vi "lv2012 - Bind Shared Variables with EPICS subVI.vi"(11 "vi path":path=path "C:/Users/kvlb23/Documents/KVLB Test Area/Research/data binding/lv2012 - SubVI 2.vi") -> (0 "error out":errorcluster)   [LabVIEW 2012]
uses:
  <vilib>/variable/tagger/epicsserver/API/internal/Undeploy EPICS Server (By Ref).vi
  Labview Modules/Common/Utilities/Equal.llb/Equal - Variant.vi
  Labview Modules/Common/Utilities/Equal.llb/Equal - String.vi
  <vilib>/variable/tagger/epicsserver/API/internal/EPICSServerClass/EPICSServer.lvclass
  <vilib>/lvdsc/NI_DSC.lvlib
  <vilib>/variable/tagger/epicsserver/API/NI_EPICS_Server.lvlib
panel:
  in  "Stop Button":bool
  in  "error in (no error)":errorcluster
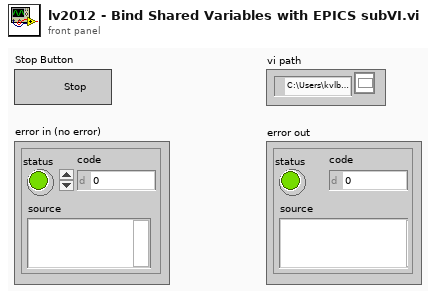
[diagram p1: front panel]
types:
  T1 = enum32{"No PSP", "Read", "Write", "Write & Read"}
  T2 = enum32{"u32BitField", "bool", "double", "string", "int8", "uint8", "int16", "uint16", "int32", "uint32", "int64", "uint64", "single", "double waveform", "int16 waveform", "array of boolean", "array of int8", "array of uint8", "array of int16", "array of uint16", "array of int32", "array of uint32", "array of int64", "array of uint64", "array of single", "array of double", "array of double waveform", "array of int16 waveform", "array of string", "variant", "timestamp", "fixed point", "custom"}
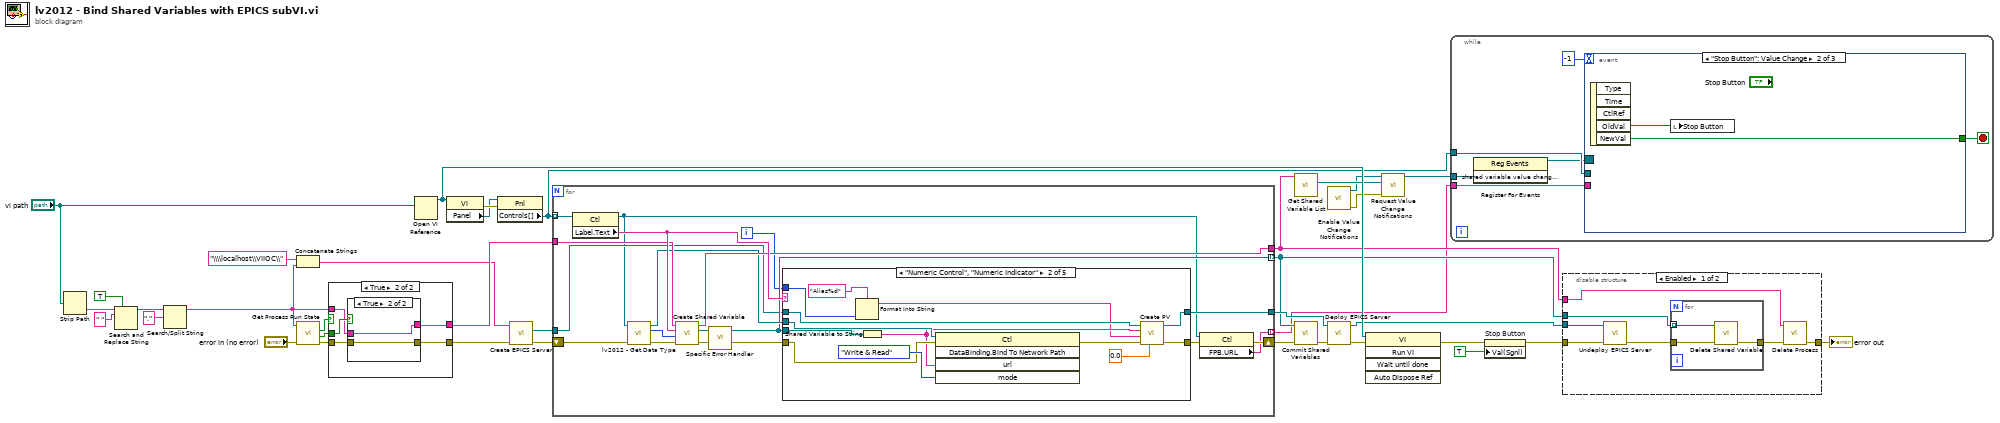
[diagram p0: block diagram]
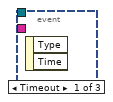
[diagram p2: hidden frame]
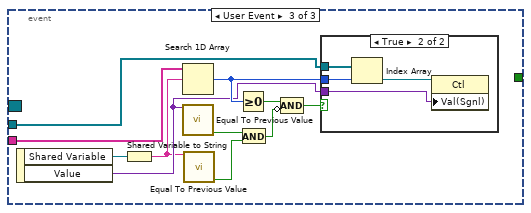
[diagram p3: hidden frame]
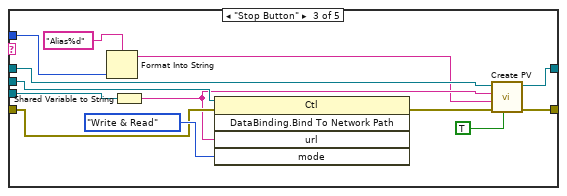
[diagram p7: hidden frame]
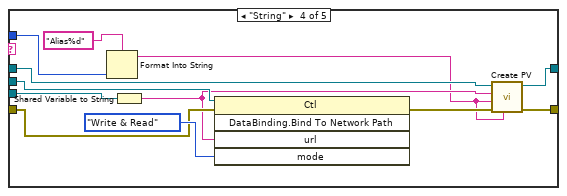
[diagram p8: hidden frame]
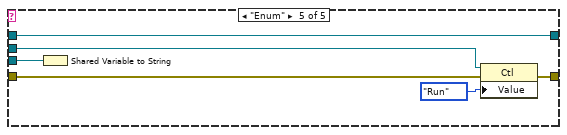
[diagram p9: hidden frame]
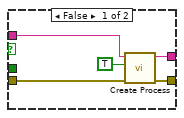
[diagram p10: hidden frame]
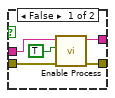
[diagram p11: hidden frame]
diagram:
  n1 = Strip Path(path="vi path") -> (name=w17:string)  [unwired: 1 out]
  n2 = Search and Replace String(replace all?=TRUE ("replace all? (F)"), input string=w17, search string=" ") -> (result string=w14:string)  [unwired: 5 in, 3 out]
  n3 = Search/Split String(string=w14, search string/char (-)="." ("regular expression")) -> (substring before match=w12:string)  [unwired: 1 in, 2 out]
  n4 = Concatenate Strings("\\\\localhost\\VIIOC\\" ("format string"), w12) -> (w18:string)
  n5 = call <vilib>:"Get Process Run State.vi"("error in (no error)"="error in (no error)", "process name"=w12) -> ("error out"=w34:errorcluster, "running?"=w33:bool, "exists?"=w36:bool)  [unwired: 6 in, 1 out]
  n6 = case shown="True" w36 {
    tunnel: w12 -> [w42 w46]
    tunnel: [w39 w44] -> w29
    tunnel: w34 -> [w41 w45]
    tunnel: [w38 w43] -> w27
    tunnel: w33 -> [_ w47]
    frame False {
      n7 = call <vilib>:"Create Process.vi"("error in (no error)"=w41, "run?"=TRUE, "process name"=w42) -> ("error out"=w38:errorcluster, "process name out"=w39:string)  [unwired: 7 in]
    }
    frame True {
      n8 = case shown="True" w47 {
        tunnel: w46 -> [w51 w54]
        tunnel: w45 -> [w50 w53]
        tunnel: [w49 w54] -> w44
        tunnel: [w48 w53] -> w43
        frame False {
          n9 = call <vilib>:"Enable Process.vi"("error in (no error)"=w50, "run?"=TRUE, "process name"=w51) -> ("error out"=w48:errorcluster, "process name out"=w49:string)  [unwired: 7 in]
        }
        frame True {
        }
      }
    }
  }
  n10 = Open VI Reference(vi path="vi path") -> (vi reference=w30:refnum<vi>)  [unwired: 5 in, 1 out]
  n11 = property class="VI"(reference=w30) -> (error out=w32:errorcluster, "Panel"=w31:refnum<vi>)  [unwired: 1 in, 1 out]
  n12 = property class="Pnl"(reference=w31, error in=w32) -> ("Controls[]"=w6:refnum<vi>[])  [unwired: 2 out]
  n13 = call <vilib>:"Create EPICS Server.vi"("error in (no error)"=w27, "EPICS Server URL in"=w18) -> ("error out"=w26:errorcluster, "EPICS Server ref"=w25:refnum<data-value>)  [unwired: 7 in, 1 out]
  n14 = for {
    tunnel: w6 -> [w72] mode=indexing
    shift-right: [w57] -> w22
    shift-left: w26 -> [w67]
    tunnel: w29 -> [w70]
    tunnel: [w69] -> w7
    tunnel: [w63] -> w23 mode=indexing
    tunnel: [w61] -> w28
    tunnel: w25 -> [w62]
    tunnel: [w55] -> w5 mode=indexing
    i -> [w60]
    n15 = property class="Ctl"(reference=w72) -> (reference out=w56:refnum<vi>, "Label.Text"=w71:string)  [unwired: 1 in, 1 out]
    n16 = call "lv2012 - Get Data Type.vi"("error in (no error)"=w67, "Control in"=w56) -> ("error out"=w66:errorcluster, "data type"=w65:T2, "Control out"=w64:refnum<vi>)  [unwired: 7 in]
    n17 = call <vilib>:"Create Shared Variable.vi"("error in (no error)"=w66, "data type"=w65, "shared variable name"=w71, "process name"=w70) -> ("error out"=w59:errorcluster, "shared variable"=w63:refnum<k21>, "process name out"=w69:string)  [unwired: 5 in]
    n18 = call "Specific Error Handler"("Error to Check"=w59) -> ("error out"=w68:errorcluster)  [unwired: 11 in, 3 out]
    n19 = case shown="\"Numeric Control\", \"Numeric Indicator\"" w71 {
      tunnel: w64 -> [_ w86 w99 w111 w116]
      tunnel: [w74 w81 w94 w106 w118] -> w58
      tunnel: w68 -> [w74 w85 w98 w110 w117]
      tunnel: w63 -> [_ w80 w93 w105 w113]
      tunnel: w62 -> [w73 w84 w97 w109 w114]
      tunnel: [w73 w83 w96 w108 w114] -> w61
      tunnel: w60 -> [_ w77 w91 w103 _]
      frame Default {
      }
      frame "Numeric Control", "Numeric Indicator" {
        n20 = Format Into String(format string="Alias%d", w77) -> (resulting string=w75:string)  [unwired: 2 in, 1 out]
        n21 = Shared Variable to String(1:w80) -> (0:w79:string)
        n22 = invoke on="Invoke Node" class="Ctl" method="DataBinding.Bind To Network Path"(reference=w86, error in=w85, "url"=w79, "mode"=T1."Write & Read" ("Data Binding:Mode")) -> (error out=w82:errorcluster)  [unwired: 1 in, 4 out]
        n23 = call <vilib>:"Create PV.vi"("data type"=0.0, "error in (no error)"=w82, "PV name"=w75, "variable path"=w79, "EPICS Server ref in"=w84) -> ("error out"=w81:errorcluster, "EPICS Server ref out"=w83:refnum<data-value>)  [unwired: 5 in]
      }
      frame "Stop Button" {
        n24 = Format Into String(format string="Alias%d", w91) -> (resulting string=w88:string)  [unwired: 2 in, 1 out]
        n25 = Shared Variable to String(1:w93) -> (0:w92:string)
        n26 = invoke on="Invoke Node" class="Ctl" method="DataBinding.Bind To Network Path"(reference=w99, error in=w98, "url"=w92, "mode"=T1."Write & Read" ("Data Binding:Mode")) -> (error out=w95:errorcluster)  [unwired: 1 in, 4 out]
        n27 = call <vilib>:"Create PV.vi"("data type"=TRUE, "error in (no error)"=w95, "PV name"=w88, "variable path"=w92, "EPICS Server ref in"=w97) -> ("error out"=w94:errorcluster, "EPICS Server ref out"=w96:refnum<data-value>)  [unwired: 5 in]
      }
      frame "String" {
        n28 = Format Into String(format string="Alias%d", w103) -> (resulting string=w101:string)  [unwired: 2 in, 1 out]
        n29 = Shared Variable to String(1:w105) -> (0:w104:string)
        n30 = invoke on="Invoke Node" class="Ctl" method="DataBinding.Bind To Network Path"(reference=w111, error in=w110, "url"=w104, "mode"=T1."Write & Read" ("Data Binding:Mode")) -> (error out=w107:errorcluster)  [unwired: 1 in, 4 out]
        n31 = call <vilib>:"Create PV.vi"("data type"=w101, "error in (no error)"=w107, "PV name"=w101, "variable path"=w104, "EPICS Server ref in"=w109) -> ("error out"=w106:errorcluster, "EPICS Server ref out"=w108:refnum<data-value>)  [unwired: 5 in]
      }
      frame "Enum" {
        n32 = Shared Variable to String(1:w113) -> ()  [unwired: 1 out]
        n33 = property class="Ctl"(reference=w116, error in=w117, "Value"=enum16{"Init", "Run", "End"}."Run" ("Enum")) -> (error out=w118:errorcluster)  [unwired: 1 out]
      }
    }
    n34 = property class="Ctl"(reference=w56, error in=w58) -> (error out=w57:errorcluster, "FPB.URL"=w55:string)  [unwired: 1 out]
  }
  n35 = call <vilib>:"Get Shared Variable List.vi"("process name"=w7) -> ("shared variables"=w9:refnum<k21>[])  [unwired: 1 in, 9 out]
  n36 = call <vilib>:"Commit Shared Variables.vi"("error in (no error)"=w22, "shared variables"=w23) -> ("error out"=w21:errorcluster)  [unwired: 8 in, 1 out]
  n37 = call <vilib>:"Enable Value Change Notifications.vi"() -> ("error out"=w10:errorcluster, "shared variable value change notification"=w8:refnum<user-event>)  [unwired: 10 in]
  n38 = call <vilib>:"Deploy EPICS Server.vi"("error in (no error)"=w21, "EPICS Server ref in"=w28) -> ("error out"=w11:errorcluster, "EPICS Server ref out"=w24:refnum<data-value>)  [unwired: 8 in]
  n39 = invoke class="VI" method="Run VI"(reference=w30, error in=w11) -> (error out=w3:errorcluster)  [unwired: 3 in, 4 out]
  n40 = call <vilib>:"Request Value Change Notifications.vi"("error in (no error)"=w10, "shared variables"=w9, "notification refnum"=w8) -> ("shared variable value change notification"=w4:refnum<user-event>)  [unwired: 6 in, 2 out]
  n41 = while {
    tunnel: w5 -> [w123]
    tunnel: w6 -> [w122]
    tunnel: w4 -> [w119]
    stop <- w121 stop-if-true
    n42 = register-events(w119) -> (reference out=w120:refnum<event-registration>)  [unwired: 2 in, 1 out]
    n43 = event shown="[1] \"Stop Button\": Value Change" {
      selector: w120 -> [_ _ _]
      dyn-events: _ -> [_ _ _]
      timeout: -1 -> [_ _ _]
      tunnel: w123 -> [_ _ w135]
      tunnel: w122 -> [_ _ w134]
      tunnel: [_ w125 _] -> w121
      event Timeout {
        n44 = event-data() -> ()  [unwired: 1 in, 2 out]
      }
      event "Stop Button": Value Change {
        n45 = event-data() -> ("OldVal"=w126:bool, "NewVal"=w125:bool)  [unwired: 1 in, 3 out]
        n46 = local write "Stop Button"(w126) -> ()
      }
      event User Event {
        n47 = event-data() -> ("Shared Variable"=w137:refnum<k21>, "Value"=w132:variant)  [unwired: 1 in]
        n48 = Shared Variable to String(1:w137) -> (0:w130:string)
        n49 = Search 1D Array(1D array=w135, element=w130) -> (index of element=w133:i32)  [unwired: 1 in]
        n50 = call-poly "Equal To Previous Value.vi"("Value In"=w132) -> ("Equal to previous value"=w129:bool)  [unwired: 13 in, 1 out]
        n51 = call-poly "Equal To Previous Value.vi"("Value In"=w130) -> ("Equal to previous value"=w128:bool)  [unwired: 13 in, 1 out]
        n52 = Greater Or Equal To 0?(x=w133) -> (x >= 0?=w136:bool)
        n53 = And(x=w129, y=w128) -> (x .and. y?=w127:bool)
        n54 = Compound Arithmetic op=AND(w136, invert w127) -> (w131:bool)
        n55 = case shown="True" w131 {
          tunnel: w134 -> [_ w141]
          tunnel: w133 -> [_ w140]
          tunnel: w132 -> [_ w138]
          frame False {
          }
          frame True {
            n56 = Index Array(array=w141, index=w140) -> (element=w139:refnum<vi>)
            n57 = property class="Ctl"(reference=w139, "Val(Sgnl)"=w138) -> ()  [unwired: 1 in, 2 out]
          }
        }
      }
    }
  }
  n58 = property on="Stop Button" class="Bool (strict)"(error in=w3, "Val(Sgnl)"=TRUE) -> (error out=w2:errorcluster)  [unwired: 1 in, 1 out]
  n59 = disable-structure shown="Enabled" {
    disable-tunnel: w7 -> [w147 _]
    disable-tunnel: w24 -> [w146 _]
    disable-tunnel: w23 -> [w145 _]
    disable-tunnel: w2 -> [w144 _]
    disable-tunnel: [w142 _] -> w20
    frame Enabled {
      n60 = call-poly <vilib>:"Undeploy EPICS Server.vi"("error in (no error)"=w144, "EPICS Server ref"=w146) -> ("error out"=w143:errorcluster)  [unwired: 9 in]
      n61 = for {
        tunnel: w145 -> [w150] mode=indexing
        tunnel: [w151] -> w148
        tunnel: w143 -> [w149]
        n62 = call <vilib>:"Delete Shared Variable.vi"("error in (no error)"=w149, "shared variable"=w150) -> ("error out"=w151:errorcluster)  [unwired: 9 in]
      }
      n63 = call <vilib>:"Delete Process.vi"("error in (no error)"=w148, "process name"=w147) -> ("error out"=w142:errorcluster)  [unwired: 9 in]
    }
    frame Disabled {
    }
  }
  "error out" <- w20
